vi "MoveForwards.vi"(0 "object in":refnum<class "Snake.lvclass">, 5 "error in (no error)":errorcluster) -> (14 "object out":refnum<class "Snake.lvclass">, 16 "New Head":T1, 17 "Deleted Tail":T1, 19 "error out":errorcluster)   [LabVIEW 2021, in "Snake.lvclass"]
uses:
  Snake.lvclass
  Coordinates.ctl
  Snake.lvclass/Snake.ctl
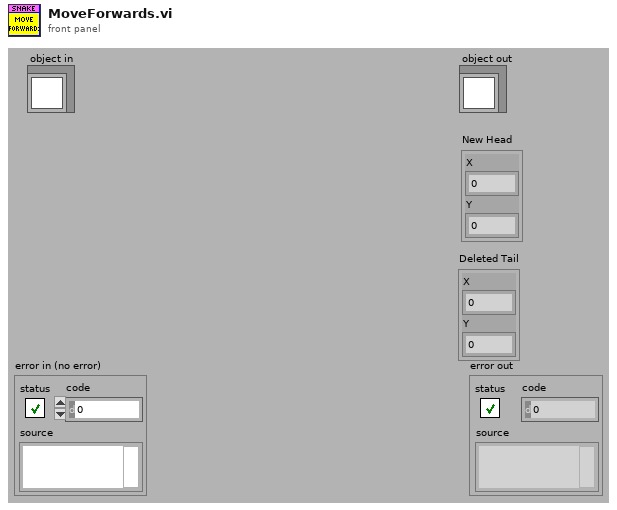
[diagram p1: front panel]
types:
  T1 = typedef "Coordinates.ctl" = cluster{"X":i32, "Y":i32}
  T2 = typedef "Direction.ctl" = enum16{"up", "down", "left", "right"}
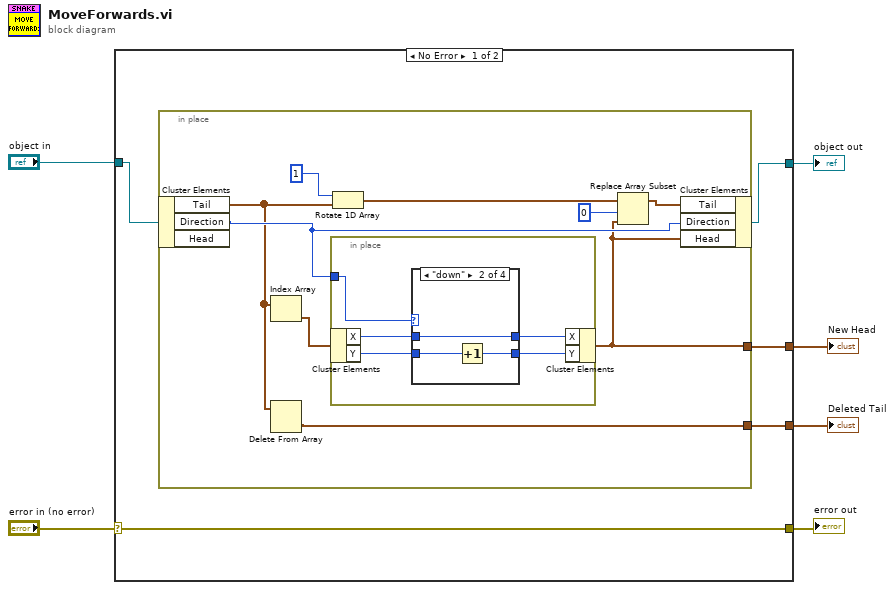
[diagram p0: block diagram]
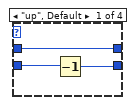
[diagram p2: hidden frame]
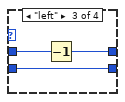
[diagram p3: hidden frame]
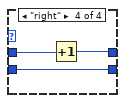
[diagram p4: hidden frame]
diagram:
  n1 = case shown="No Error" "error in (no error)" {
    selector: "error in (no error)" -> [w11 w39]
    tunnel: [w11 w39] -> w5
    tunnel: [w8 w38] -> w3
    tunnel: "object in" -> [w10 w38]
    tunnel: [w9 _] -> w2
    tunnel: [w7 _] -> w1
    frame No Error {
      n2 = in-place {
        in-place-border: [w13] -> w9
        in-place-border: [w12] -> w7
        n3 = in-place-cluster #1(w10) -> ("Tail"=w14:T1[], "Direction"=w16:T2)  [unwired: 1 out]
        n4 = Index Array(array=w14) -> (element=w17:T1)  [unwired: 1 in]
        n5 = Delete From Array(array=w14) -> (deleted portion=w13:T1)  [unwired: 2 in, 1 out]
        n6 = in-place {
          in-place-border: w16 -> [w25]
          n7 = in-place-cluster #2(w17) -> ("X"=w24:i32, "Y"=w23:i32)
          n8 = case shown="\"down\"" w25 {
            tunnel: w24 -> [w26 w29 w34 w37]
            tunnel: w23 -> [w28 w31 w32 w35]
            tunnel: [w27 w30 w32 w35] -> w22
            tunnel: [w26 w29 w33 w36] -> w21
            frame "up", Default {
              n9 = Decrement(x=w28) -> (x-1=w27:i32)
            }
            frame "down" {
              n10 = Increment(x=w31) -> (x+1=w30:i32)
            }
            frame "left" {
              n11 = Decrement(x=w34) -> (x-1=w33:i32)
            }
            frame "right" {
              n12 = Increment(x=w37) -> (x+1=w36:i32)
            }
          }
          n13 = in-place-cluster #2("X"=w21, "Y"=w22) -> (w12:T1)
        }
        n14 = Rotate 1D Array(1:w14, 2:1 ("n")) -> (0:w20:T1[])
        n15 = Replace Array Subset(array=w20, new element=w12, index=0) -> (w19:T1[])
        n16 = in-place-cluster #1("Tail"=w19, "Direction"=w16, "Head"=w12) -> (w8:refnum<class "Snake.lvclass">)
      }
    }
    frame Error {
    }
  }
  "error out" <- w5
  "object out" <- w3
  "New Head" <- w1
  "Deleted Tail" <- w2
